vi "IIR Notch Peak Filter Design.vi"() -> ()   [LabVIEW 2023]
doc: "Demonstrates how to use the DFD IIR Notch Peak Design VI to design different types of notch/peak filters with different sets of parameters.\n\nComplete the following steps to use this VI.\n1) Run the VI.\n2) Set the <B>Filter Type</B> to <B>Notch</B> or <B>Peak</B>.\n3) View the By Q-factor or By Bandwidth page and change the parameters.\n4) Observe the Magnitude Squared graph.\n5) Switch to the other page and try the other set of parameters.\n6) Observe the Magnitude Squared graph.\n7) Click the <B>STOP</B> button to stop this VI."
uses:
  <vilib>/addons/Digital Filter Design/Design.llb/DFD IIR Notch Peak Design by Q.vi
  <vilib>/addons/Digital Filter Design/Design.llb/DFD IIR Notch Peak Design by BW.vi
  <vilib>/addons/Digital Filter Design/Analysis.llb/DFD Plot Freq Response (Linear-Spaced).vi
  <vilib>/addons/Digital Filter Design/NI_DigFilterLicensed.lvlib
panel:
  in  "stop":bool
  out "Error Message":string
  in  "Design Method":enum32{"By Q-factor", "By Bandwidth"}(tab)=enum."By Bandwidth"
  in  "Q factor":dbl=25.0 format="%.2f"
  in  "Ab [dB]":dbl=3.010299956639812 format="%#.6g"
  in  "Bandwidth [Hz]":dbl=8.0 format="%.2f"
  out "Magnitude Squared":cluster{"f0":dbl, "df":dbl, "values":dbl[]}(graph)
  in  "fs [Hz]":dbl=1000.0 format="%.2f"
  in  "f0 [Hz]":dbl=200.0 format="%.2f"
  in  "Filter Type":u16(ring) items=["Notch", "Peak"]
  # "Select Help>>Show Context Help and move the cursor over the VI icon for more information."
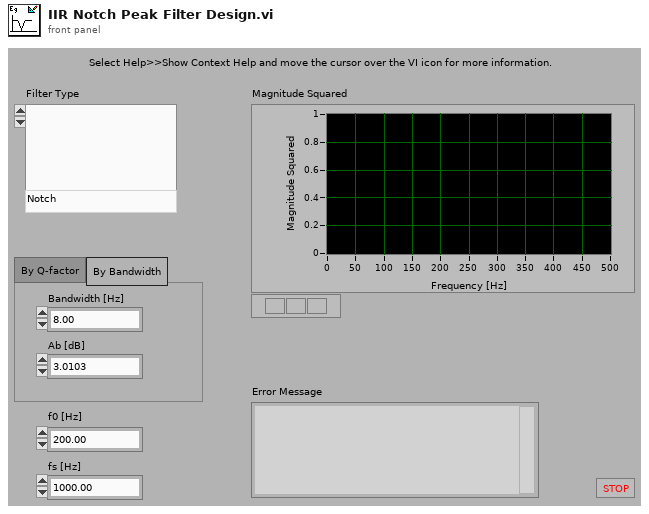
[diagram p1: front panel]
types:
  T1 = typedef "NI_DigFilterLicensed.lvlib/DFD Filter Obj.ctl" = cluster{"mSRate_Fs":dbl, "mSRate_Version":string, "mSRate_Comments":string, "mSRate_OrgCoef":T2, "mSRate_CurCoef":T2, "mSRate_Quantized?":bool, "mSRate_QCoef":T2, "mSRate_QSettings":T4[], "mSRate_Order":i32, "mSRate_Scaling":cluster{"mSRate_ScaleByPowerOf2?":bool, "mSRate_ScaleType":T6}}
  T2 = typedef "NI_DigFilterLicensed.lvlib/DFD Filter Coef.ctl" = cluster{"type":T3, "gain":dbl, "coef a (k)":dbl[], "coef b (v)":dbl[]}
  T3 = typedef "NI_DigFilterLicensed.lvlib/DFD Filter Structure Type Selector.ctl" = enum16{"Undefined", "FIR Direct Form", "FIR Direct Form Transposed", "FIR Symmetric", "FIR Antisymmetric", "IIR Direct Form I", "IIR Direct Form I Transposed", "IIR Direct Form II", "IIR Direct Form II Transposed", "IIR Cascaded Second Order Sections Form I", "IIR Cascaded Second Order Sections Form I Transposed", "IIR Cascaded Second Order Sections Form II", "IIR Cascaded Second Order Sections Form II Transposed", "Lattice Allpass (basic sections)", "Lattice Allpass (one multiplier sections)", "Lattice Allpass (normalized sections)", "Lattice AR (basic sections)", "Lattice AR (one multiplier sections)", "Lattice AR (normalized sections)", "Lattice MA (minimum phase)", "Lattice MA (maximum phase)", "Lattice ARMA (basic sections)", "Lattice ARMA (one multiplier sections)", "Lattice ARMA (normalized sections)"}
  T4 = typedef "NI_DigFilterLicensed.lvlib/dfd_Internal Quantization Settings.ctl" = cluster{"source":T5, "wl":i16, "iwl":i16, "overflow mode":enum16{"Saturation", "Wrap"}, "rounding mode":enum16{"Nearest", "Truncation"}, "signed?":bool}
  T5 = typedef "NI_DigFilterLicensed.lvlib/dfd_Internal Quantization Srcs.ctl" = u16
  T6 = typedef "NI_DigFilterLicensed.lvlib/DFD Coef Norm Type.ctl" = enum16{"No Norm", "Time Domain 1-Norm", "Time Domain 2-Norm", "Time Domain Inf-Norm"}
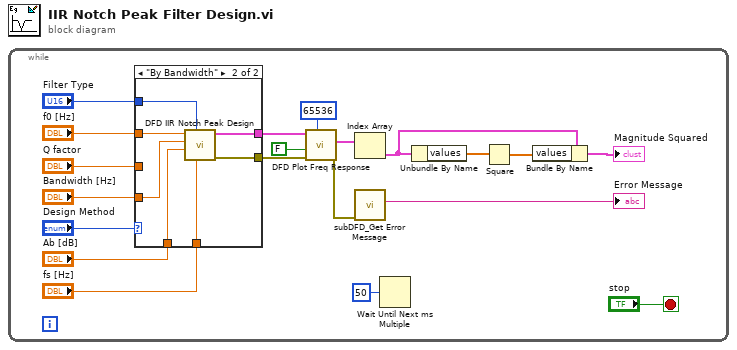
[diagram p0: block diagram]
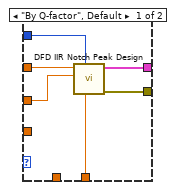
[diagram p2: hidden frame]
diagram:
  n1 = while {
    stop <- "stop" stop-if-true
    n2 = case shown="\"By Bandwidth\"" "Design Method" {
      tunnel: "Q factor" -> [w23 _]
      tunnel: "Bandwidth [Hz]" -> [_ w30]
      tunnel: "f0 [Hz]" -> [w26 w33]
      tunnel: "Filter Type" -> [w24 w32]
      tunnel: [w25 w31] -> w16
      tunnel: "Ab [dB]" -> [_ w29]
      tunnel: "fs [Hz]" -> [w22 w28]
      tunnel: [w21 w27] -> w15
      frame "By Q-factor", Default {
        n3 = call-poly <vilib>:"DFD IIR Notch Peak Design.vi"("fs [Hz]"=w22, "filter type"=w24, "Q factor"=w23, "f0 [Hz]"=w26) -> ("error out"=w21:errorcluster, "filter out"=w25:T1)  [unwired: 1 in, 5 out]
      }
      frame "By Bandwidth" {
        n4 = call-poly <vilib>:"DFD IIR Notch Peak Design.vi"("fs [Hz]"=w28, "filter type"=w32, "Ab [dB]"=w29, "Df [Hz]"=w30, "f0 [Hz]"=w33) -> ("error out"=w27:errorcluster, "filter out"=w31:T1)  [unwired: 1 in, 4 out]
      }
    }
    n5 = call-poly <vilib>:"DFD Plot Freq Response.vi"("# freq bins"=65536 ("# freq bins (auto)"), "error in (no error)"=w15, "dB on? (T)"=FALSE, "filter in"=w16) -> ("error out"=w12:errorcluster, "magnitude response"=w4:cluster{"f0":dbl, "df":dbl, "values":dbl[]}[])  [unwired: 4 in, 2 out]
    n6 = Index Array(array=w4) -> (element=w14:cluster{"f0":dbl, "df":dbl, "values":dbl[]})  [unwired: 1 in]
    n7 = call <vilib>:"subDFD_Get Error Message.vi"("error in (no error)"=w12) -> ("Error Message"=→"Error Message":string)  [unwired: 10 out]
    n8 = Wait Until Next ms Multiple(millisecond multiple=u32 50) -> ()  [unwired: 1 out]
    n9 = Unbundle By Name(w14) -> ("values"=w2:dbl[])
    n10 = Square(x=w2) -> (x^2=w1:dbl[])
    n11 = Bundle By Name(cluster=w14, "values"=w1) -> (→"Magnitude Squared":cluster{"f0":dbl, "df":dbl, "values":dbl[]})
  }
